vi "Strings.vi"() -> ()   [LabVIEW 2018]
panel:
  in  "Search String":string
  out "Final String":string
  out "Resultant String":string
  out "Length":i32
  in  "Replace String":string
  out "Length":i32
  in  "Input String":string
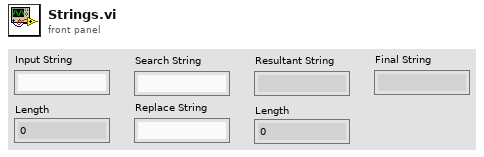
[diagram p1: front panel]
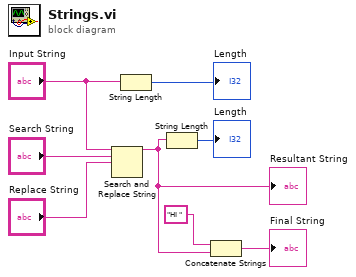
[diagram p0: block diagram]
diagram:
  n1 = Search and Replace String(input string="Input String", search string="Search String", replace string="Replace String") -> (result string=w1:string)  [unwired: 5 in, 3 out]
  "Resultant String" <- w1
  n2 = String Length(string="Input String") -> (length=→"Length":i32)
  n3 = String Length(string=w1) -> (length=→"Length":i32)
  n4 = Concatenate Strings("HI ", w1) -> (→"Final String":string)
